vi "Retriggerable Acquisition DAQ.vi"() -> ()   [LabVIEW 2020]
uses:
  <vilib>/DAQmx/read.llb/DAQmx Read (Analog 1D DBL 1Chan NSamp).vi
  <vilib>/DAQmx/create/channels.llb/DAQmx Create Channel (AI-Voltage-Basic).vi
  <vilib>/DAQmx/configure/timing.llb/DAQmx Timing (Sample Clock).vi
  <vilib>/DAQmx/configure/trigger.llb/DAQmx Start Trigger (Digital Edge).vi
  <vilib>/DAQmx/miscellaneous.llb/DAQmx Fill In Error Info.vi
panel:
  in  "stop":bool
  in  "edge":i32(ring)=10280 items=["Rising"=10280, "Falling"=10171]
  in  "source":tag
  out "Waveform Graph":dbl[](graph)
  in  "rate":dbl=1000.0 format="%0.2f"
  in  "samples per channel":i32=1000
  in  "sample mode":i32(ring)=10178 items=["Finite Samples"=10178, "Continuous Samples"=10123, "Hardware Timed Single Point"=12522]
  in  "physical channels":tag
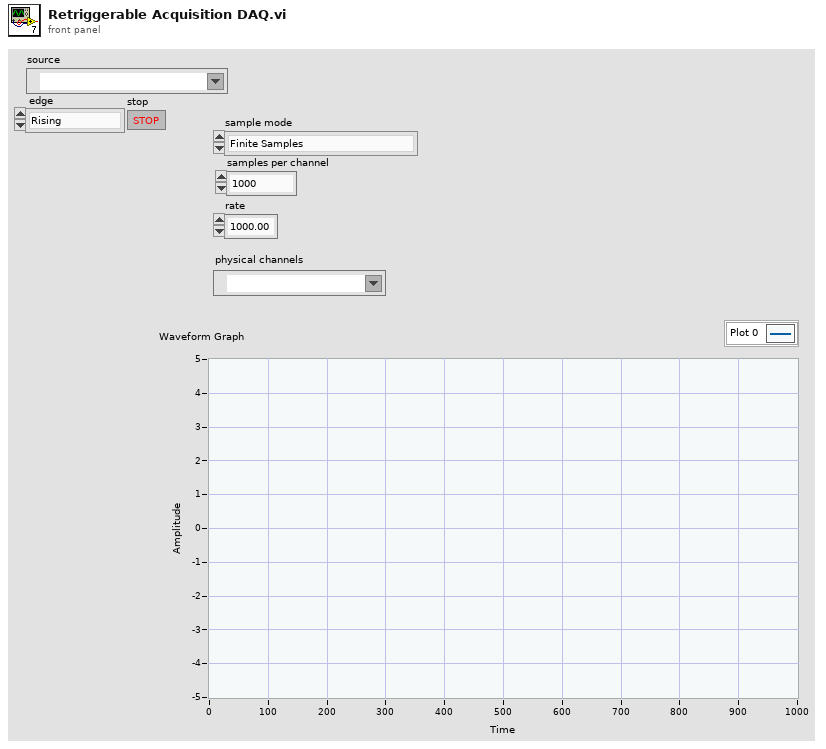
[diagram p1: front panel]
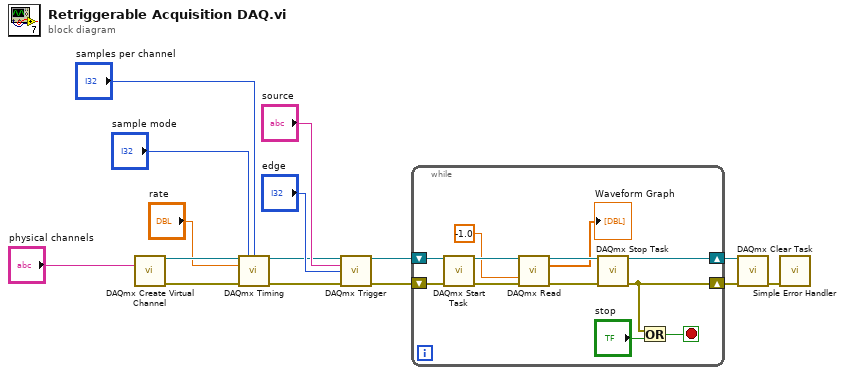
[diagram p0: block diagram]
diagram:
  n1 = call-poly <vilib>:"DAQmx Create Virtual Channel.vi"("physical channels"="physical channels") -> ("task out"=w14:refnum<k21>, "error out"=w13:errorcluster)  [unwired: 13 in]
  n2 = call-poly <vilib>:"DAQmx Timing.vi"("task/channels in"=w14, "sample mode"="sample mode", "samples per channel"="samples per channel", "rate"="rate", "error in"=w13) -> ("task out"=w4:refnum<k21>, "error out"=w3:errorcluster)  [unwired: 9 in]
  n3 = call-poly <vilib>:"DAQmx Trigger.vi"("task/channels in"=w4, "source"="source", "edge"="edge", "error in"=w3) -> ("task out"=w2:refnum<k21>, "error out"=w1:errorcluster)  [unwired: 10 in]
  n4 = while {
    shift-right: [w19] -> w9
    shift-left: w2 -> [w17]
    shift-right: [w18] -> w8
    shift-left: w1 -> [w16]
    stop <- w20 stop-if-true
    n5 = call <vilib>:"DAQmx Start Task.vi"("task/channels in"=w17, "error in"=w16) -> ("task out"=w27:refnum<k21>, "error out"=w26:errorcluster)  [unwired: 12 in]
    n6 = call-poly <vilib>:"DAQmx Read.vi"("task/channels in"=w27, "timeout"=-1.0, "error in"=w26) -> ("task out"=w25:refnum<k21>, "data"=→"Waveform Graph":dbl[], "error out"=w24:errorcluster)  [unwired: 10 in]
    n7 = call <vilib>:"DAQmx Stop Task.vi"("task/channels in"=w25, "error in"=w24) -> ("task out"=w19:refnum<k21>, "error out"=w18:errorcluster)  [unwired: 12 in]
    n8 = Or(x=w18, y="stop") -> (x .or. y?=w20:bool)
  }
  n9 = call <vilib>:"DAQmx Clear Task.vi"("task in"=w9, "error in"=w8) -> ("error out"=w7:errorcluster)  [unwired: 13 in]
  n10 = call <vilib>:"Simple Error Handler.vi"("error in (no error)"=w7) -> ()  [unwired: 4 in, 5 out]
